vi "Pin Name.vi"() -> (2 "pin name":string="niDCPower")   [LabVIEW 2021, in "Converter Reusables.lvlib"]
uses:
  Converter Reusables.lvlib
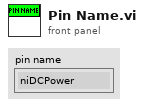
[diagram p1: front panel]
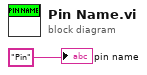
[diagram p0: block diagram]
diagram:
  "pin name" <- "Pin" ("Pin Name")
